vi "Post-Build Action.vi"(5 "Files Generated by Build":path[](array[path]), 6 "Top Level/Always Included VIs":path[](array[path]), 7 "Destination Path":path, 8 "error in (no error)":errorcluster, 9 "Target Name":string, 10 "Build Specification Name":string, 11 "Project Path":path) -> (0 "error out":errorcluster)   [LabVIEW 2014]
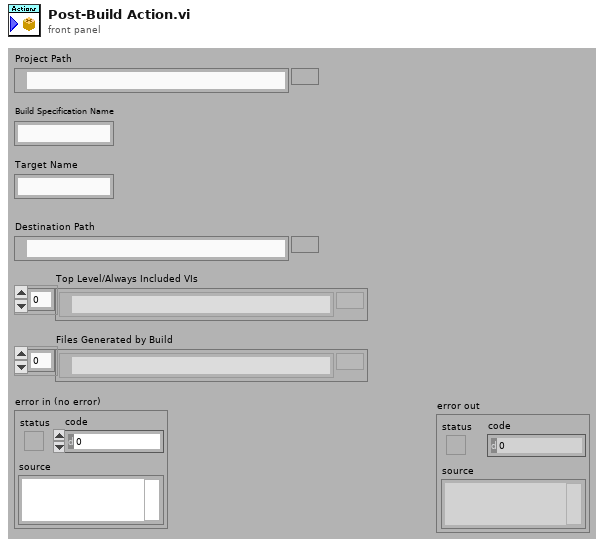
[diagram p1: front panel]
types:
  T1 = enum16{"open", "replace", "create", "open or create", "replace or create", "replace or create with confirmation"}
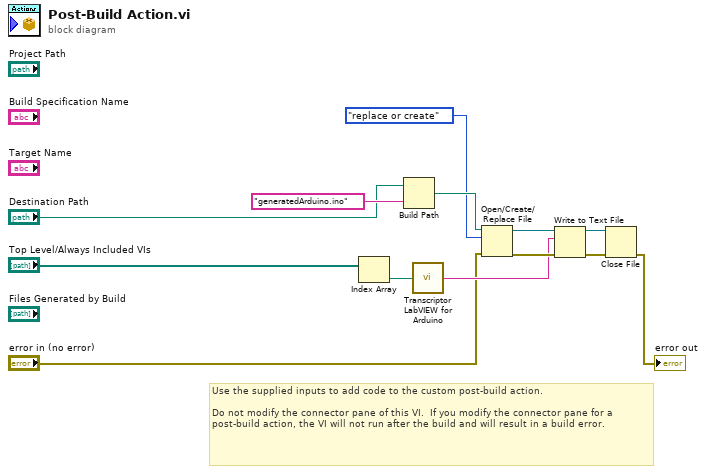
[diagram p0: block diagram]
diagram:
  # "Use the supplied inputs to add code to the custom post-build action.\n\nDo not modify the connector pane of this VI.  If you modify the connector pane for a post-build action, the VI will not run after the build and will result in a build error."
  n1 = Index Array(array="Top Level/Always Included VIs") -> (element=w12:path)  [unwired: 1 in]
  n2 = Build Path(base path="Destination Path", name or relative path="generatedArduino.ino") -> (appended path=w11:path)
  n3 = call <vilib>:"Transcriptor LabVIEW for Arduino.vi"("vi path"=w12) -> ("transcripted code"=w9:string)
  n4 = Open/Create/Replace File(file path (use dialog)=w11, error in="error in (no error)", operation (0:open)=T1."replace or create") -> (refnum out=w8:refnum<file>, error out=w10:errorcluster)  [unwired: 3 in, 1 out]
  n5 = Write to Text File(file (use dialog)=w8, text=w9, error in=w10) -> (refnum out=w5:refnum<file>, error out=w6:errorcluster)  [unwired: 1 in, 1 out]
  n6 = Close File(refnum=w5, error in=w6) -> (error out=→"error out":errorcluster)  [unwired: 1 out]
